vi "ActiveObject_QueueQueue_ProcessRepository_EndevoGoop3.vi"(0 "reference in":refnum<class>, 1 "Action(ReadRepository)":T1(ring), 5 "error in (no error)":errorcluster) -> (9 "ProcessViRef":refnum<vi>, 11 "ProcessSyncQueue":refnum<queue>, 13 "FromProcessQueue":refnum<queue>, 14 "reference out":refnum<class>, 15 "ToProcessQueue":refnum<queue>, 17 "ProcessAlreadyStarted":bool, 19 "error out":errorcluster)   [LabVIEW 2016]
uses:
  <resource>/Framework/Providers/Open_GDS/ClassProviders/DesignPatterns/ActiveObjects/ActiveObjects_QueueQueue_SubVIs/ActiveObject_QueueQueue_Process.ctl
panel:
  # "Use this indicator for sending messages to the Process VI"
  # "These indicators are used by the process VIs"
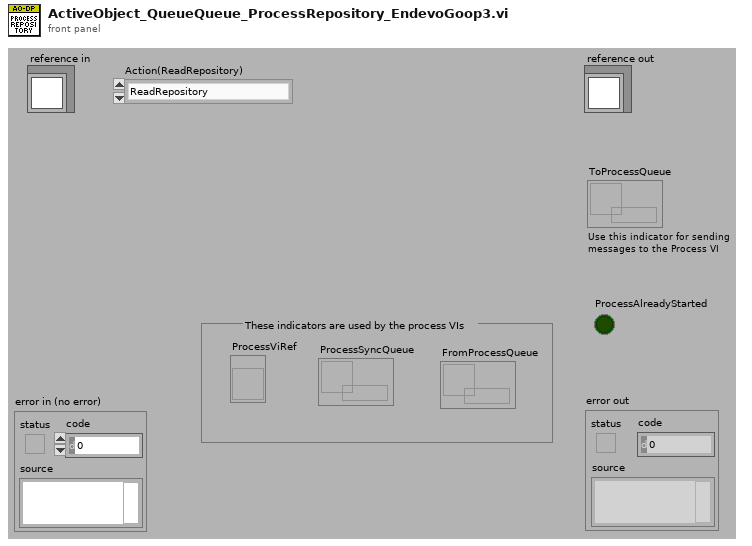
[diagram p1: front panel]
types:
  T1 = enum16{"ReadRepository", "CreateNew", "CreateOrLookUpExisting", "ReadRepositoryAndDestroy"}
  T2 = typedef "ActiveObject_QueueQueue_Process.ctl" = cluster{"ToProcessQueue":refnum<queue>, "FromProcessQueue":refnum<queue>, "ProcessSyncQueue":refnum<queue>, "ProcessViRef":refnum<vi>}
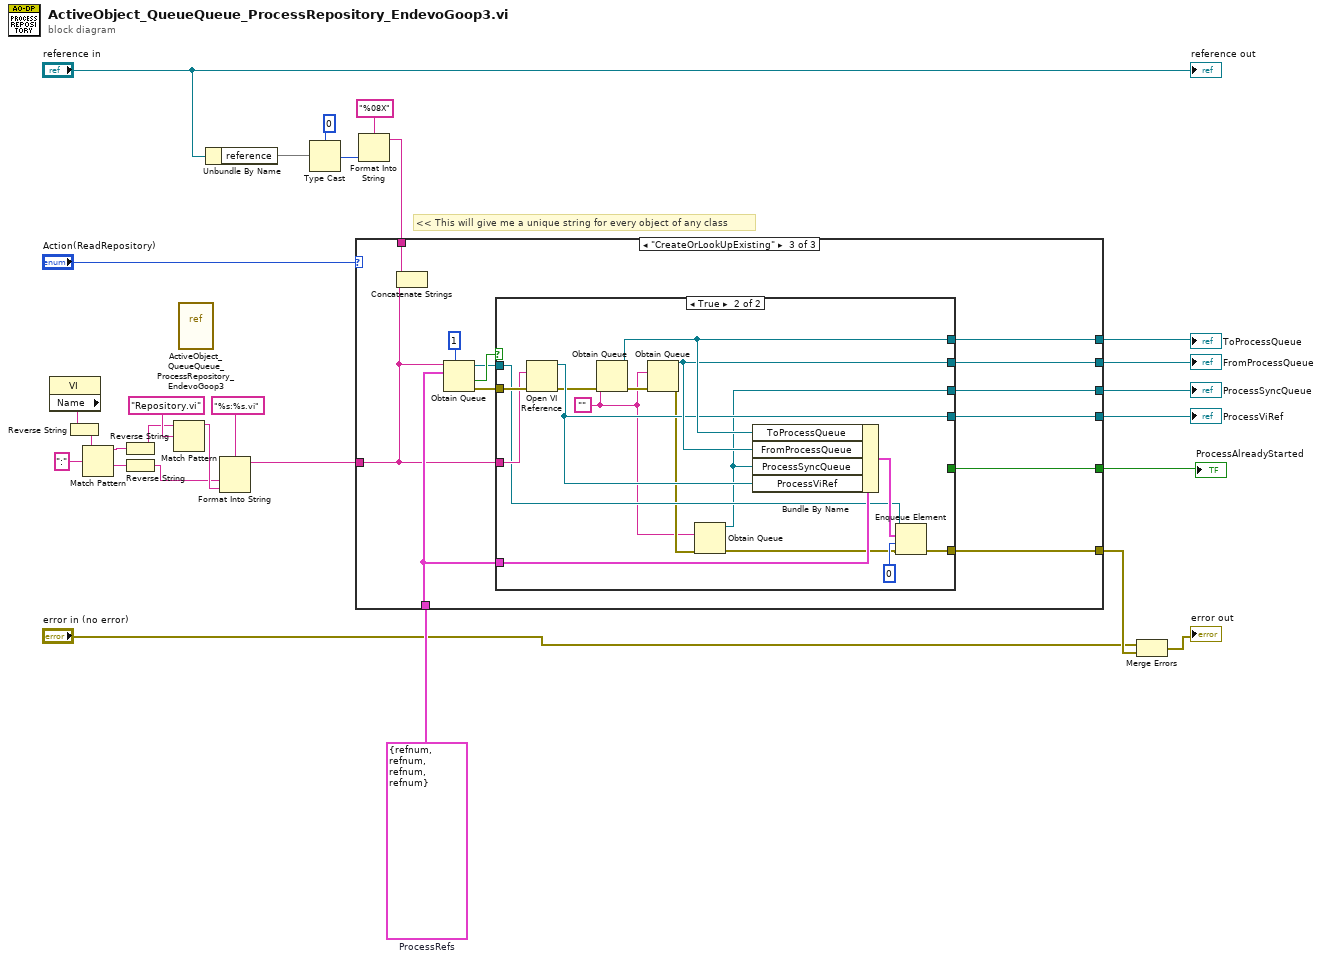
[diagram p0: block diagram]
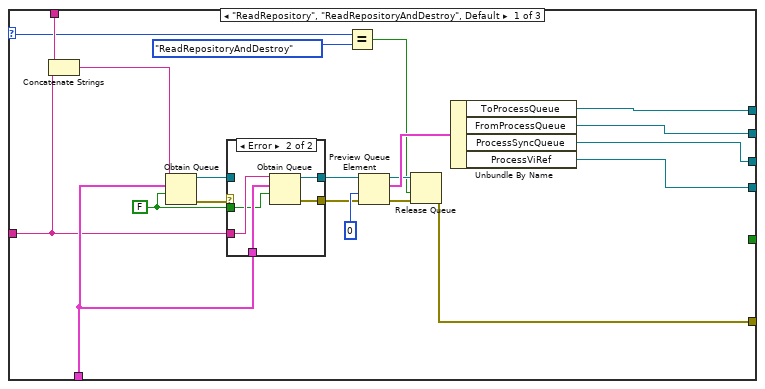
[diagram p2: hidden frame]
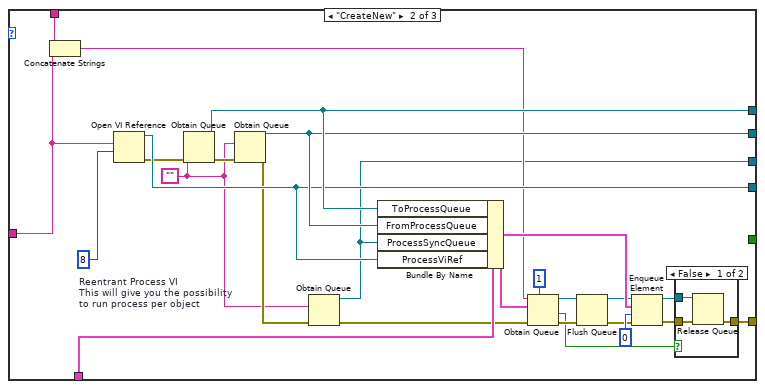
[diagram p4: hidden frame]
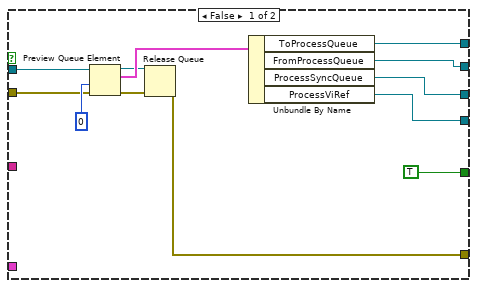
[diagram p6: hidden frame]
diagram:
  w22 = T2 {"ToProcessQueue"=refnum, "FromProcessQueue"=refnum, "ProcessSyncQueue"=refnum, "ProcessViRef"=refnum}  # ProcessRefs
  # "<< This will give me a unique string for every object of any class"
  n1 = property class="VI"() -> ("Name"=w11:string)  [unwired: 2 in, 2 out]
  n2 = Reverse String(1:w11) -> (0:w12:string)
  n3 = Match Pattern(string=w12, regular expression=":") -> (before substring=w16:string, after substring=w13:string)  [unwired: 1 in, 2 out]
  n4 = Reverse String(1:w16) -> (0:w17:string)
  n5 = Reverse String(1:w13) -> (0:w15:string)
  n6 = Match Pattern(string=w17, regular expression="Repository.vi") -> (before substring=w19:string)  [unwired: 1 in, 3 out]
  n7 = vi-ref <resource>:"ActiveObject_QueueQueue_ProcessRepository_EndevoGoop3.vi"() -> ()  [unwired: 1 out]
  n8 = Unbundle By Name("reference in") -> ("reference"=w1)
  n9 = Format Into String(format string="%s:%s.vi", w15, w19) -> (resulting string=w9:string)  [unwired: 2 in, 1 out]
  n10 = Type Cast(type=u32 0, x=w1) -> (*(type *) &x=w6:u32)
  n11 = Format Into String(format string="%08X", w6) -> (resulting string=w3:string)  [unwired: 2 in, 1 out]
  n12 = case shown="\"CreateOrLookUpExisting\"" "Action(ReadRepository)" {
    selector: "Action(ReadRepository)" -> [w29 _ _]
    tunnel: [w43 w64 w95] -> w26
    tunnel: [w45 w80 w97] -> w24
    tunnel: [w44 w79 w96] -> w25
    tunnel: [w46 w78 w94] -> w23
    tunnel: w22 -> [w38 w70 w90]
    tunnel: w3 -> [w36 w69 w86]
    tunnel: [w31 w57 w93] -> w20
    tunnel: w9 -> [w35 w67 w85]
    tunnel: [_ _ w88] -> w8
    frame "ReadRepository", "ReadRepositoryAndDestroy", Default {
      w37 = FALSE ("create if not found? (T)")
      n13 = Concatenate Strings(w36, w35) -> (w34:string)
      n14 = Obtain Queue(name (unnamed)=w34, element data type=w38, create if not found? (T)=w37) -> (queue out=w40:refnum<queue>, error out=w42:errorcluster)  [unwired: 2 in, 1 out]
      n15 = case shown="Error" w42 {
        selector: w42 -> [w50 _]
        tunnel: [w50 w52] -> w41
        tunnel: w40 -> [w49 _]
        tunnel: [w49 w53] -> w39
        tunnel: w38 -> [_ w55]
        tunnel: w35 -> [_ w54]
        tunnel: w37 -> [_ w51]
        frame No Error {
        }
        frame Error {
          n16 = Obtain Queue(name (unnamed)=w54, element data type=w55, create if not found? (T)=w51) -> (queue out=w53:refnum<queue>, error out=w52:errorcluster)  [unwired: 2 in, 1 out]
        }
      }
      n17 = Equal?(x=w29, y=T1."ReadRepositoryAndDestroy") -> (x = y?=w28:bool)
      n18 = Preview Queue Element(queue=w39, timeout in ms (-1)=0, error in (no error)=w41) -> (queue out=w33:refnum<queue>, element=w47:T2, error out=w32:errorcluster)  [unwired: 1 out]
      n19 = Release Queue(queue=w33, force destroy? (F)=w28, error in (no error)=w32) -> (error out=w31:errorcluster)  [unwired: 2 out]
      n20 = Unbundle By Name(w47) -> ("ToProcessQueue"=w45:refnum<queue>, "FromProcessQueue"=w44:refnum<queue>, "ProcessSyncQueue"=w43:refnum<queue>, "ProcessViRef"=w46:refnum<vi>)
    }
    frame "CreateNew" {
      w75 = 8  # Reentrant Process VI This will give you the possibility to run process per object
      w63 = ""
      n21 = Concatenate Strings(w69, w67) -> (w68:string)
      n22 = Open VI Reference(vi path=w67, options=w75) -> (vi reference=w78:refnum<vi>, error out=w76:errorcluster)  [unwired: 4 in]
      n23 = Obtain Queue(element data type=w63, error in (no error)=w76) -> (queue out=w80:refnum<queue>, error out=w77:errorcluster)  [unwired: 3 in, 1 out]
      n24 = Obtain Queue(element data type=w63, error in (no error)=w77) -> (queue out=w79:refnum<queue>, error out=w66:errorcluster)  [unwired: 3 in, 1 out]
      n25 = Obtain Queue(element data type=w63, error in (no error)=w66) -> (queue out=w64:refnum<queue>, error out=w65:errorcluster)  [unwired: 3 in, 1 out]
      n26 = Bundle By Name(cluster=w70, "ToProcessQueue"=w80, "FromProcessQueue"=w79, "ProcessSyncQueue"=w64, "ProcessViRef"=w78) -> (w73:T2)
      n27 = Obtain Queue(max queue size (-1, unlimited)=1, name (unnamed)=w68, element data type=w73, error in (no error)=w65) -> (queue out=w74:refnum<queue>, created new?=w56:bool, error out=w61:errorcluster)  [unwired: 1 in]
      n28 = Flush Queue(queue=w74, error in (no error)=w61) -> (queue out=w62:refnum<queue>, error out=w60:errorcluster)  [unwired: 1 out]
      n29 = Enqueue Element(queue=w62, element=w73, timeout in ms (-1)=0, error in (no error)=w60) -> (queue out=w59:refnum<queue>, error out=w58:errorcluster)  [unwired: 1 out]
      n30 = case shown="False" w56 {
        tunnel: w58 -> [w83 w84]
        tunnel: w59 -> [w82 _]
        tunnel: [w81 w84] -> w57
        frame False {
          n31 = Release Queue(queue=w82, error in (no error)=w83) -> (error out=w81:errorcluster)  [unwired: 1 in, 2 out]
        }
        frame True {
        }
      }
    }
    frame "CreateOrLookUpExisting" {
      n32 = Concatenate Strings(w86, w85) -> ()  [unwired: 1 out]
      n33 = Obtain Queue(max queue size (-1, unlimited)=1, name (unnamed)=w85, element data type=w90) -> (queue out=w91:refnum<queue>, created new?=w92:bool, error out=w89:errorcluster)  [unwired: 2 in]
      n34 = case shown="True" w92 {
        tunnel: [w109 w125] -> w97
        tunnel: [w108 w124] -> w96
        tunnel: [w107 w110] -> w95
        tunnel: [w106 w123] -> w94
        tunnel: [w98 w122] -> w93
        tunnel: w90 -> [_ w121]
        tunnel: w89 -> [w103 w116]
        tunnel: w85 -> [_ w115]
        tunnel: w91 -> [w104 w114]
        tunnel: [TRUE _] -> w88
        frame False {
          n35 = Preview Queue Element(queue=w104, timeout in ms (-1)=0, error in (no error)=w103) -> (queue out=w100:refnum<queue>, element=w102:T2, error out=w99:errorcluster)  [unwired: 1 out]
          n36 = Release Queue(queue=w100, error in (no error)=w99) -> (error out=w98:errorcluster)  [unwired: 1 in, 2 out]
          n37 = Unbundle By Name(w102) -> ("ToProcessQueue"=w109:refnum<queue>, "FromProcessQueue"=w108:refnum<queue>, "ProcessSyncQueue"=w107:refnum<queue>, "ProcessViRef"=w106:refnum<vi>)
        }
        frame True {
          w111 = ""
          n38 = Open VI Reference(vi path=w115, error in (no error)=w116) -> (vi reference=w123:refnum<vi>, error out=w119:errorcluster)  [unwired: 4 in]
          n39 = Obtain Queue(element data type=w111, error in (no error)=w119) -> (queue out=w125:refnum<queue>, error out=w120:errorcluster)  [unwired: 3 in, 1 out]
          n40 = Obtain Queue(element data type=w111, error in (no error)=w120) -> (queue out=w124:refnum<queue>, error out=w113:errorcluster)  [unwired: 3 in, 1 out]
          n41 = Obtain Queue(element data type=w111, error in (no error)=w113) -> (queue out=w110:refnum<queue>, error out=w112:errorcluster)  [unwired: 3 in, 1 out]
          n42 = Bundle By Name(cluster=w121, "ToProcessQueue"=w125, "FromProcessQueue"=w124, "ProcessSyncQueue"=w110, "ProcessViRef"=w123) -> (w118:T2)
          n43 = Enqueue Element(queue=w114, element=w118, timeout in ms (-1)=0, error in (no error)=w112) -> (error out=w122:errorcluster)  [unwired: 2 out]
        }
      }
    }
  }
  "ProcessSyncQueue" <- w26
  "ToProcessQueue" <- w24
  "FromProcessQueue" <- w25
  "ProcessViRef" <- w23
  "ProcessAlreadyStarted" <- w8
  n44 = Merge Errors("error in (no error)", w20) -> (→"error out":errorcluster)
  "reference out" <- "reference in"
